vi "r_item_insert.vi"(6 "ms timeout (0:default)":i32, 7 "db":string, 8 "error in (no error)":errorcluster, 9 "json":string, 10 "table":string, 11 "rethinkdb in":T1) -> (0 "error out":errorcluster, 1 "response":variant, 2 "generated_keys":string[](array[string]), 3 "rethinkdb out":T1)   [LabVIEW 2017, in "rethinkdb.lvlib"]
uses:
  rethinkdb.lvlib
  refnum.ctl
  ql2_term.ctl
  ql2_query.ctl
  4facdf79-eaab-4117-9226-3fa19dc40407.vi
  ql2_term_to_id.vi
  ql2_query_to_id.vi
  json_get_names.vi
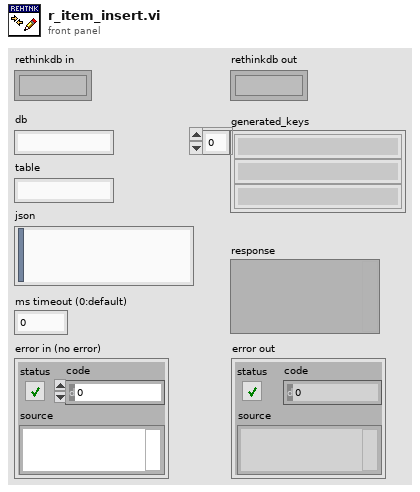
[diagram p1: front panel]
types:
  T1 = typedef "rethinkdb.lvlib/refnum.ctl" = refnum<k1>
  T2 = typedef "rethinkdb.lvlib/ql2_term.ctl" = enum8{"ADD", "AND", "APPEND", "APRIL", "ARGS", "ASC", "AUGUST", "AVG", "BETWEEN", "BETWEEN_DEPRECATED", "BINARY", "BIT_AND", "BIT_NOT", "BIT_OR", "BIT_SAL", "BIT_SAR", "BIT_XOR", "BRACKET", "BRANCH", "CEIL", "CHANGES", "CHANGE_AT", "CIRCLE", "COERCE_TO", "CONCAT_MAP", "CONFIG", "CONTAINS", "COUNT", "DATE", "DATUM", "DAY", "DAY_OF_WEEK", "DAY_OF_YEAR", "DB", "DB_CREATE", "DB_DROP", "DB_LIST", "DECEMBER", "DEFAULT", "DELETE", "DELETE_AT", "DESC", "DIFFERENCE", "DISTANCE", "DISTINCT", "DIV", "DOWNCASE", "DURING", "EPOCH_TIME", "EQ", "EQ_JOIN", "ERROR", "FEBRUARY", "FILL", "FILTER", "FLOOR", "FOLD", "FOR_EACH", "FRIDAY", "FUNC", "FUNCALL", "GE", "GEOJSON", "GET", "GET_ALL", "GET_FIELD", "GET_INTERSECTING", "GET_NEAREST", "GET_WRITE_HOOK", "GRANT", "GROUP", "GT", "HAS_FIELDS", "HOURS", "HTTP", "IMPLICIT_VAR", "INCLUDES", "INDEX_CREATE", "INDEX_DROP", "INDEX_LIST", "INDEX_RENAME", "INDEX_STATUS", "INDEX_WAIT", "INFO", "INNER_JOIN", "INSERT", "INSERT_AT", "INTERSECTS", "IN_TIMEZONE", "ISO8601", "IS_EMPTY", "JANUARY", "JAVASCRIPT", "JSON", "JULY", "JUNE", "KEYS", "LE", "LIMIT", "LINE", "LITERAL", "LT", "MAKE_ARRAY", "MAKE_OBJ", "MAP", "MARCH", "MATCH", "MAX", "MAXVAL", "MAY", "MERGE", "MIN", "MINUTES", "MINVAL", "MOD", "MONDAY", "MONTH", "MUL", "NE", "NOT", "NOVEMBER", "NOW", "NTH", "OBJECT", "OCTOBER", "OFFSETS_OF", "OR", "ORDER_BY", "OUTER_JOIN", "PLUCK", "POINT", "POLYGON", "POLYGON_SUB", "PREPEND", "RANDOM", "RANGE", "REBALANCE", "RECONFIGURE", "REDUCE", "REPLACE", "ROUND", "SAMPLE", "SATURDAY", "SECONDS", "SEPTEMBER", "SET_DIFFERENCE", "SET_INSERT", "SET_INTERSECTION", "SET_UNION", "SET_WRITE_HOOK", "SKIP", "SLICE", "SPLICE_AT", "SPLIT", "STATUS", "SUB", "SUM", "SUNDAY", "SYNC", "TABLE", "TABLE_CREATE", "TABLE_DROP", "TABLE_LIST", "THURSDAY", "TIME", "TIMEZONE", "TIME_OF_DAY", "TO_EPOCH_TIME", "TO_GEOJSON", "TO_ISO8601", "TO_JSON_STRING", "TUESDAY", "TYPE_OF", "UNGROUP", "UNION", "UPCASE", "UPDATE", "UUID", "VALUES", "VAR", "WAIT", "WEDNESDAY", "WITHOUT", "WITH_FIELDS", "YEAR", "ZIP", "invalid"}
  T3 = typedef "rethinkdb.lvlib/ql2_query.ctl" = enum8{"START", "CONTINUE", "STOP", "NOREPLY_WAIT", "SERVER_INFO", "invalid"}
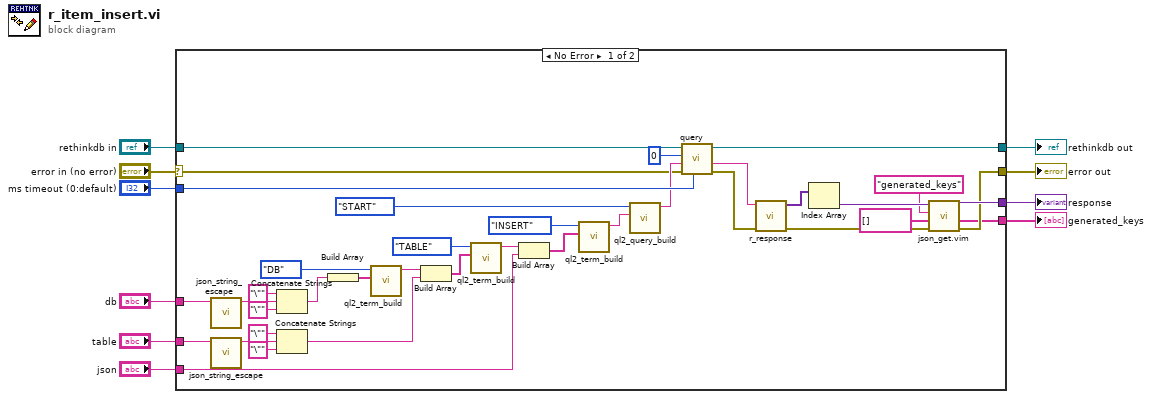
[diagram p0: block diagram]
diagram:
  n1 = case shown="No Error" "error in (no error)" {
    selector: "error in (no error)" -> [w23 w49]
    tunnel: "rethinkdb in" -> [w24 w48]
    tunnel: [w47 w48] -> w8
    tunnel: "ms timeout (0:default)" -> [w46 _]
    tunnel: [w14 w49] -> w6
    tunnel: "db" -> [w45 _]
    tunnel: [w15 _] -> w4
    tunnel: "table" -> [w44 _]
    tunnel: "json" -> [w18 _]
    tunnel: [w12 _] -> w1
    frame No Error {
      n2 = call "json_string_escape.vi"("string"=w45) -> ("escaped string"=w32:string)  [unwired: 10 in]
      n3 = call "json_string_escape.vi"("string"=w44) -> ("escaped string"=w43:string)  [unwired: 10 in]
      n4 = Concatenate Strings("\"" ("string"), w32, "\"" ("string")) -> (w29:string)
      n5 = Concatenate Strings("\"" ("string"), w43, "\"" ("string")) -> (w25:string)
      n6 = Build Array(w29) -> (w35:string[])
      n7 = call "ql2_term_build.vi"("args"=w35, "term_type"=ql2_term."DB") -> ("query"=w34:string)  [unwired: 9 in]
      n8 = Build Array(w34, w25) -> (w33:string[])
      n9 = call "ql2_term_build.vi"("args"=w33, "term_type"=ql2_term."TABLE") -> ("query"=w21:string)  [unwired: 9 in]
      n10 = Build Array(w21, w18) -> (w20:string[])
      n11 = call "ql2_term_build.vi"("args"=w20, "term_type"=ql2_term."INSERT") -> ("query"=w19:string)  [unwired: 9 in]
      n12 = call "ql2_query_build.vi"("query"=w19, "query_type"=ql2_query."START") -> ("query"=w41:string)  [unwired: 9 in]
      n13 = call "query.vi"("ms timeout (0:default)"=w46, "error in (no error)"=w23, "query"=w41, "token in (random)"=u64 0, "rethinkdb in"=w24) -> ("error out"=w40:errorcluster, "response"=w39:string, "rethinkdb out"=w47:T1)  [unwired: 3 in, 1 out]
      n14 = call "r_response.vi"("error in (no error)"=w40, "response"=w39) -> ("error out"=w17:errorcluster, "values"=w28:variant[])  [unwired: 8 in]
      n15 = Index Array(array=w28) -> (element=w16:variant)  [unwired: 1 in]
      n16 = call "json_get.vim"("error in (no error)"=w17, "default"=string[] [], "name"="generated_keys", "variant in"=w16) -> ("error out"=w14:errorcluster, "value"=w12:string[], "variant out"=w15:variant)  [unwired: 4 in, 1 out]
    }
    frame Error {
    }
  }
  "error out" <- w6
  "rethinkdb out" <- w8
  "response" <- w4
  "generated_keys" <- w1
